vi "Shutdown.vi"(8 "error in":errorcluster) -> (0 "error out":errorcluster)   [LabVIEW 2020, in "Hardware.lvlib"]
uses:
  Hardware.lvlib
  Messaging/Message FGV Actions.ctl
panel:
  # "Message Handler: Shutdown"
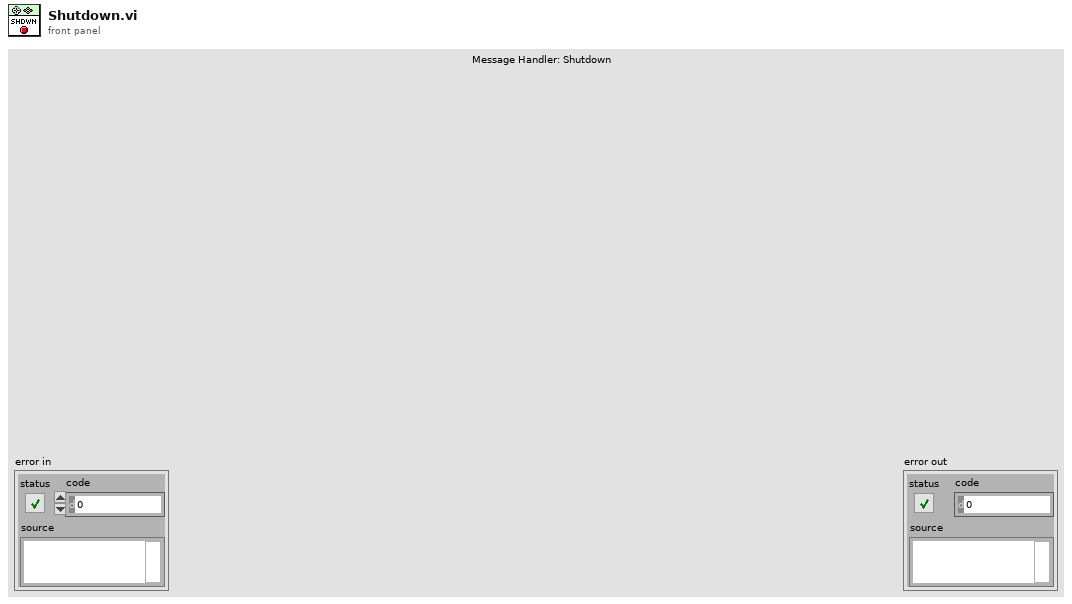
[diagram p1: front panel]
types:
  T1 = typedef "Hardware.lvlib/Message FGV Actions.ctl" = enum16{"Get", "Obtain", "Release", "Flush"}
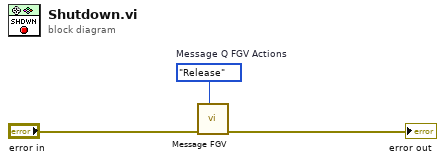
[diagram p0: block diagram]
diagram:
  w3 = Message_FGV_Actions."Release"  # Message Q FGV Actions
  n1 = call "Message FGV.vi"("Message Q FGV Actions"=w3, "error in"="error in") -> ("error out"=→"error out":errorcluster)  [unwired: 6 in, 3 out]
